vi "Info.vi"(11 "Nav Route in":refnum<class "Nav Route.lvclass">) -> (0 "Styles":map{string, string}(c390), 1 "Classes":set{string}(c389), 2 "Path":string, 3 "Label":string)   [LabVIEW 2020, in "Volatus.lvlib" / "Nav Route.lvclass"]
uses:
  Nav Route.lvclass
  Nav Route.lvclass/Nav Route.ctl
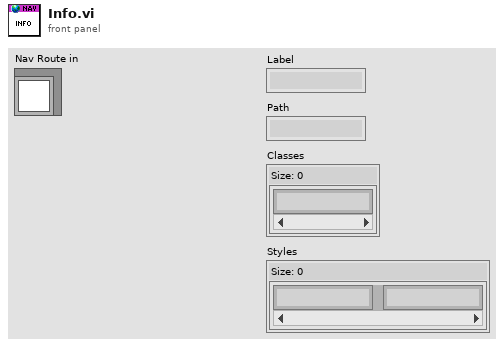
[diagram p1: front panel]
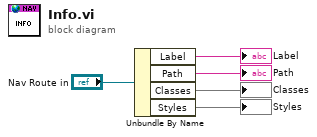
[diagram p0: block diagram]
diagram:
  n1 = Unbundle By Name("Nav Route in") -> ("Label"=→"Label":string, "Path"=→"Path":string, "Classes"=→"Classes":set{string}, "Styles"=→"Styles":map{string, string})
